vi "Write and Read Multiple Registers Request.vi"(4 "Quantity to Read":u16, 6 "Read Starting Address":u16, 8 "error in":errorcluster, 9 "Write":u16[](array[numeric]), 10 "Write Starting Address":u16) -> (0 "error out":errorcluster, 2 "modbus data unit out":refnum<class "Modbus Data Unit.lvclass">)   [LabVIEW 2021, in "Master Function Definition.lvclass"]
doc: "This VI forms a modbus data unit for simultaneously reading and writing multiple registers."
uses:
  Master Function Definition.lvclass
  Modbus Data Unit/Modbus Data Unit.lvclass
  Modbus Data Unit/Function.ctl
  Modbus Data Unit/Modbus Data Unit.lvclass/Modbus Data Unit.ctl
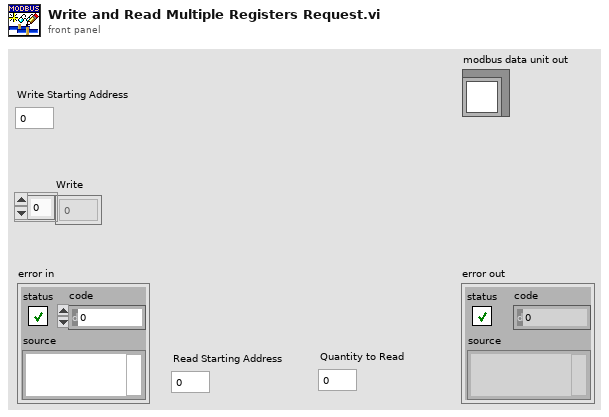
[diagram p1: front panel]
types:
  T1 = typedef "Modbus Data Unit.lvclass/Function.ctl" = u8
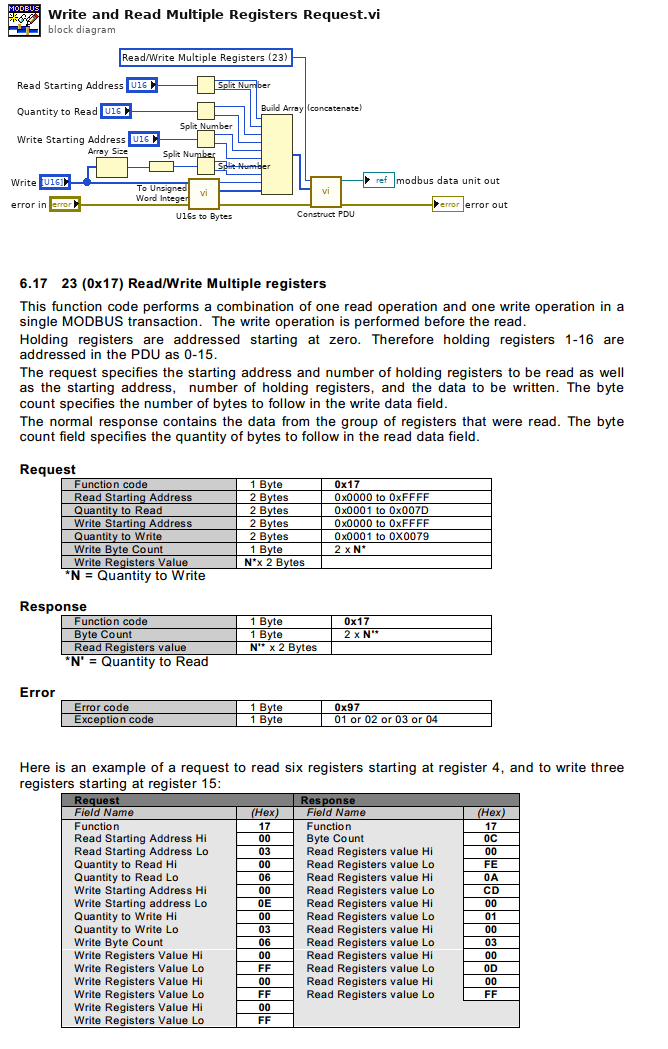
[diagram p0: block diagram]
diagram:
  w12 = T1 23 items=["Read Discrete Inputs"=2, "Read Coils"=1, "Write Single Coil"=5, "Write Multiple Coils"=15, "Read Input Register"=4, "Read Holding Registers"=3, "Write Single Register"=6, "Write Multiple Registers"=16, "Read/Write Multiple Registers"=23, "Mask Write Register"=22, "Read FIFO Queue"=24, "Read File Record"=20, "Write File Record"=21, "Read Exception Status"=7, "Diagnostic"=8, "Get Com Event Counter"=11, "Get Com Event Log"=12, "Report Slave ID"=17, "Read Device Identification"=43] ("Function")
  n1 = Array Size(array="Write") -> (size(s)=w10:i32)
  n2 = To Unsigned Word Integer(number=w10) -> (unsigned 16bit integer=w9:u16)
  n3 = call "U16s to Bytes.vi"("Registers"="Write") -> ("Bytes"=w7:u8[], "Count"=w8:u8)  [unwired: 9 in]
  n4 = Split Number(x="Read Starting Address") -> (hi(x)=w1:u8, lo(x)=w2:u8)
  n5 = Split Number(x="Quantity to Read") -> (hi(x)=w3:u8, lo(x)=w4:u8)
  n6 = Split Number(x="Write Starting Address") -> (hi(x)=w14:u8, lo(x)=w15:u8)
  n7 = Split Number(x=w9) -> (hi(x)=w16:u8, lo(x)=w17:u8)
  n8 = Build Array (concatenate)(w1, w2, w3, w4, w14, w15, w16, w17, w8, w7) -> (w13:u8[])
  n9 = call "Construct PDU.vi"("error in"="error in", "data"=w13, "Function"=w12) -> ("error out"=→"error out":errorcluster, "modbus data unit out"=→"modbus data unit out":refnum<class "Modbus Data Unit.lvclass">)  [unwired: 7 in]
